vi "Create(冲突时的文件备份2013-03-27 14-07-15).vi"(8 "error in (no error)":errorcluster caption="错误输入（无错误）", 10 "driveName":string, 11 "DriveInfo 输入":refnum<class "DriveInfo.lvclass"> caption="DNL_LabVIEW Object in") -> (0 "error out":errorcluster caption="错误输出", 3 "DriveInfo 输出":refnum<class "DriveInfo.lvclass"> caption="DNL_LabVIEW Object out")   [LabVIEW 2012, in "DriveInfo.lvclass"]
uses:
  DriveInfo.lvclass
  DriveInfo.lvclass/DriveInfo.ctl
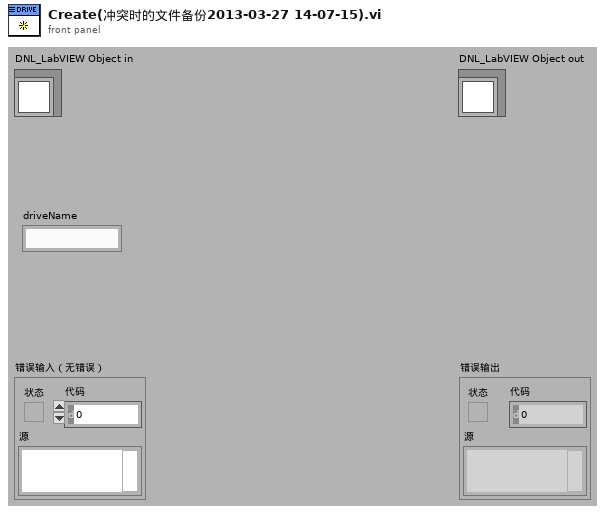
[diagram p1: front panel]
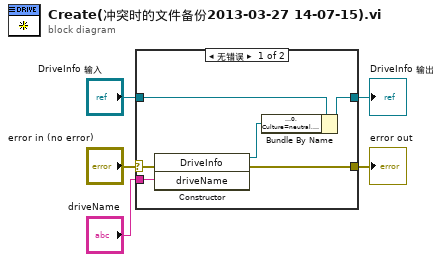
[diagram p0: block diagram]
diagram:
  n1 = case shown="无错误" "error in (no error)" {
    selector: "error in (no error)" -> [w10 w13]
    tunnel: [w6 w13] -> w4
    tunnel: [w7 w12] -> w2
    tunnel: "DriveInfo 输入" -> [w9 w12]
    tunnel: "driveName" -> [w11 _]
    frame No Error {
      n2 = constructor class="DriveInfo"(error in=w10, "driveName"=w11) -> (reference out=w8:refnum<k24>, error out=w6:errorcluster)  [unwired: 2 in, 2 out]
      n3 = Bundle By Name(cluster=w9, "DriveInfo"=w8) -> (w7:refnum<class "DriveInfo.lvclass">)
    }
    frame Error {
    }
  }
  "error out" <- w4
  "DriveInfo 输出" <- w2
